vi "Format Data to Image.vi"(5 "FFT value magnification":dbl=1000.0, 7 "#A-lines per B-line":u32=2048, 10 "Z pixels":u32=1024, 11 "data in":sgl[](array[numeric])) -> (2 "single type B-line":sgl[][](array[numeric]), 3 "U16 B-line":u16[][](array[numeric]))   [LabVIEW 2018]
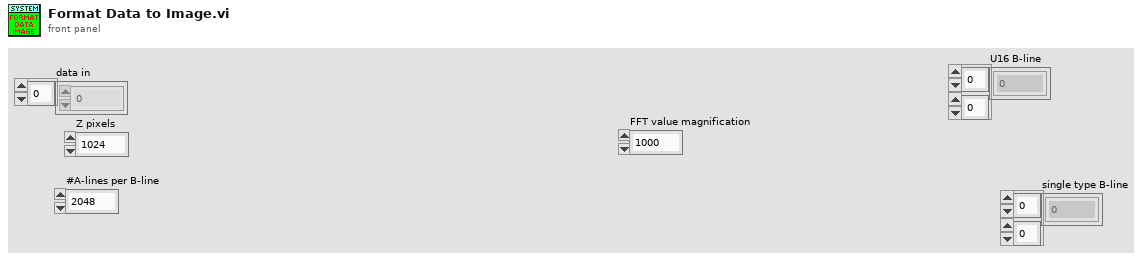
[diagram p1: front panel]
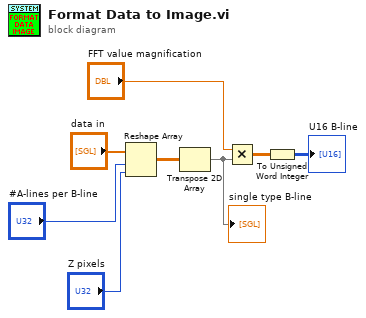
[diagram p0: block diagram]
diagram:
  n1 = Reshape Array("data in", "#A-lines per B-line", "Z pixels") -> (w5:sgl[][])
  n2 = Transpose 2D Array(2D array=w5) -> (transposed array=w3:sgl[][])
  "single type B-line" <- w3
  n3 = Multiply(x="FFT value magnification", y=w3) -> (x*y=w2:dbl[][])
  n4 = To Unsigned Word Integer(number=w2) -> (unsigned 16bit integer=→"U16 B-line":u16[][])
